vi "WriteTorqueWaveform.vi"(7 "Name":string, 8 "error in (no error)":errorcluster, 9 "Torque Waveform Unit":string, 10 "Torque Waveform":waveform(dbl), 11 "map in":T1) -> (0 "error out":errorcluster, 3 "map out":T1)   [LabVIEW 2017, in "McsaUtilities.lvlib"]
uses:
  <vilib>/addons/InsightCM/Utilities/MCSA/McsaUtilities.lvlib
  <vilib>/addons/PointValueMap/controls/PointMap.ctl
  <vilib>/addons/PointValueMap/subVIs/Point_Write_variant.vi
  <vilib>/addons/PointValueMap/PointValueMap.lvlib
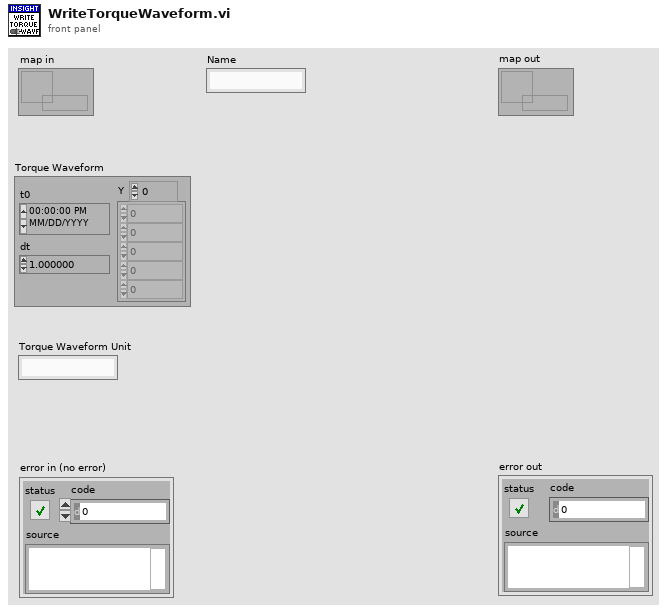
[diagram p1: front panel]
types:
  T1 = typedef "PointValueMap.lvlib/PointMap.ctl" = refnum<data-value>
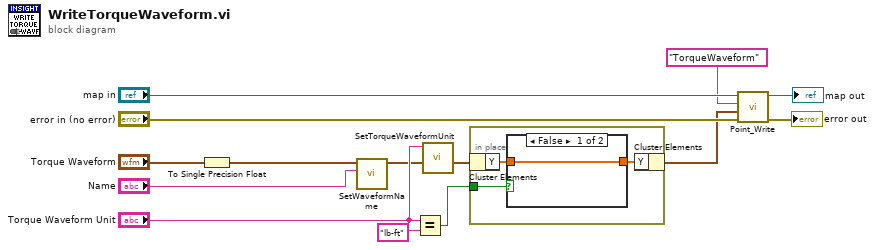
[diagram p0: block diagram]
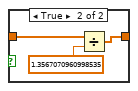
[diagram p2: hidden frame]
diagram:
  n1 = To Single Precision Float(number="Torque Waveform") -> (single precision float=w3:waveform(sgl))
  n2 = call <vilib>:"SetWaveformName.vi"("Name"="Name", "Waveform in"=w3) -> ("Waveform out"=w1:waveform(sgl))  [unwired: 8 in, 1 out]
  n3 = Equal?(x="Torque Waveform Unit", y="lb-ft") -> (x = y?=w5:bool)
  n4 = call <vilib>:"SetTorqueWaveformUnit.vi"("Waveform in"=w1, "Name"="Torque Waveform Unit") -> ("Waveform out"=w7:waveform(sgl))  [unwired: 8 in, 1 out]
  n5 = in-place {
    in-place-border: w5 -> [w15]
    n6 = in-place-cluster #1(w7) -> ("Y"=w17:sgl[])
    n7 = case shown="False" w15 {
      tunnel: w17 -> [w18 w19]
      tunnel: [w18 w21] -> w16
      frame False {
      }
      frame True {
        n8 = Divide(x=w19, y=sgl 1.3567071) -> (x/y=w21:sgl[])
      }
    }
    n9 = in-place-cluster #1("Y"=w16) -> (w6:waveform(sgl))
  }
  n10 = call-poly <vilib>:"Point_Write.vi"("Error In"="error in (no error)", "Value"=w6, "Tag"="TorqueWaveform", "Map"="map in") -> ("Error Out"=→"error out":errorcluster, "Map Out"=→"map out":T1)  [unwired: 6 in]
